vi "PROJEKT-APIR-IMIR.vi"() -> ()   [LabVIEW 2019]
uses:
  <vilib>/addons/Control Design/_Model Construction/Model Typedefs.llb/CD Transfer Function Model (MIMO).ctl
  <vilib>/addons/Control Design/_Model Construction/Model Typedefs.llb/CD General Elements.ctl
  <vilib>/addons/Control Design/_Model Construction/Model Typedefs.llb/CD Transfer Function Model (SISO).ctl
  <vilib>/addons/Control Design/_Model Construction/Data Typedefs.llb/CD MIMO Time Response Data.ctl
  <vilib>/addons/Control Design/_Model Construction/Data Typedefs.llb/CD Plot Types Enum.ctl
  <vilib>/addons/Control Design/_Model Construction/Data Typedefs.llb/CD frequency specs.ctl
  <vilib>/addons/Control Design/_Model Construction/Data Typedefs.llb/CD Time Info.ctl
  <vilib>/addons/Control Design/_Model Conversions/Model Type.llb/Model Conversion SubVI/cd_Convert Transfer Function to State-Space Model.vi
  <vilib>/addons/Control Design/_Frequency Response Analysis/Frequency Response.llb/Frequency Response subVI/cd_Bode (State Space).vi
  <vilib>/addons/Control Design/_Frequency Response Analysis/Frequency Response.llb/Frequency Response subVI/cd_Evaluate at Frequency (State-Space).vi
  <vilib>/addons/Control Design/_Frequency Response Analysis/Frequency Response.llb/Frequency Response subVI/cd_Nyquist (State-Space).vi
  <vilib>/addons/Control Design/_Model Construction/Model Creation.llb/Model Creation SubVI/cd_Create Symbolic Transfer Function Model.vi
  <vilib>/addons/Control Design/_Utility/Model Viewer.llb/Model Viewer SubVI/cd_Draw State-Space Equation (SS).vi
  <vilib>/addons/Control Design/_Utility/Model Viewer.llb/Model Viewer SubVI/cd_Draw Transfer Function Equation (TF).vi
  <vilib>/addons/Control Design/_Model Interconnection/Model Interconnection.llb/Model Interconnection SubVI/cd_Element Multiply Models (TF and Gain).vi
  <vilib>/addons/Control Design/_Time Response Analysis/Time Response.llb/Time Response subVI/cd_Initial Response (State-Space).vi
  <vilib>/addons/Control Design/_Time Response Analysis/Time Response.llb/Time Response subVI/cd_Step Response (State-Space).vi
  <vilib>/addons/Control Design/_Time Response Analysis/Time Response.llb/Time Response subVI/cd_Impulse Response (State-Space).vi
  <vilib>/addons/Control Design/_Time Response Analysis/Time Response.llb/Time Response subVI/cd_Linear Simulation (State-Space).vi
  <vilib>/addons/Control Design/_Time Response Analysis/Time Response.llb/Time Response subVI/cd_Impulse Response (Transfer Function).vi
  <vilib>/addons/Control Design/_Model Construction/NI_LinSys_Model Creation.lvlib
  <vilib>/addons/Control Design/_Utility/NI_CD_Model Viewer.lvlib
  <vilib>/addons/Control Design/_Time Response Analysis/NI_CD_Time Response.lvlib
  <vilib>/addons/Control Design/_Model Conversions/NI_CD_Model Type.lvlib
  <vilib>/addons/Control Design/_Model Construction/NI_LinSys_Data Typedefs.lvlib
  <vilib>/addons/Control Design/_Frequency Response Analysis/NI_CD_Frequency Response.lvlib
  <vilib>/addons/Control Design/_Model Interconnection/NI_CD_Model Interconnection.lvlib
  <vilib>/addons/Control Design/_Model Construction/NI_LinSys_Model Typedefs.lvlib
panel:
  in  "input cluster":T1={"Time"=array[5001 elements], "Outputs Data"=array1x5001x1[5001 elements], "States Data"=array1x5001x2[10002 elements], "plot type"=enum."impulse"} {"States Data" format="%#.6g"; "Outputs Data" format="%#.6g"; "Time" format="%#.6g"}
  in  "Initial Conditions":dbl[](array[numeric])=[0.0, 0.0]
  out "Transfer Function Model":T3={"properties"={"Model name"="System Model", "Input names"=["u0"], "Output names"=["y0"], "Input Delays"=[0.0], "Output Delays"=[0.0], "Sampling Time"=0.0, "Notes"=""}, "transfer function(s)"=[[{"Numerator"=[-1.0], "Denominator"=[3.0, 2.0, 4.0], "delay"=0.0}]]} {"transfer function(s)"."delay" format="%.4f"; "transfer function(s)"."Denominator" format="%#_3g"; "transfer function(s)"."Numerator" format="%#_3g"; "properties"."Sampling Time" format="%#.6p"; "properties"."Output Delays" format="%.4f"; "properties"."Input Delays" format="%.4f"}
  in  "Draw Area Size":cluster{"Width":u32, "Height":u32}={"Width"=117, "Height"=36}
  in  "Origin Drawing":cluster{"x":i16, "y":i16}={"x"=4, "y"=6}
  in  "y":dbl=-9.0 min=-9.0 format="%#_13g"
  in  "stop":bool
  in  "?":T6(tab)=enum."Animacja"
  in  "Masa":dbl=4.0 min=1.0 format="%#_6p"
  in  "Współczynnik tłumienia":dbl=2.0 min=1.0 format="%#_6p"
  in  "Współczynnik sprężystości":dbl=3.0 min=1.0 format="%#_6p"
  out "Equation":picture
  out "Equation 2":picture
  out "Equation 3":picture
  in  "Typ charakterystyki":u16(ring)=2 items=["All in one", "Odpowiedź na skok", "Odpowiedź na impuls", "Odpowiedź na wym. sinusoidalne", "Odpowiedź tylko na warunki początkowe"]
  in  "Siła Przyłożona \"w dół\"":dbl=-1.0 step=0.1 format="%#_6p"
  in  "Wychylenie początkowe":dbl min=0.0 step=0.1 format="%#_6p"
  in  "Prędkość początkowa":dbl min=0.0 step=0.1 format="%#_6p"
  in  "Częstotliwosć źródła":dbl=10.0 caption="Frequency" step=10.0
  out "All 2":cluster{"time":dbl[], dbl[]}[](graph)
  in  "Jednostka czestotliwosci":enum16{"Hz", "rad/s"}(ring)
  in  "Czestotliwosc poczatkowa":dbl=-1.0
  in  "Wartosc czestotliwosci":dbl=4.0 step=0.1
  out "Charakterystyka amplitudowo fazowa":cluster{"W":dbl[], "Magnitude":dbl[]}[](graph)
  out "Charakterystyka fazowo czestotliwosciowa":cluster{"W":dbl[], "Magnitude":dbl[]}[](graph)
  out "Charakterystyka amplitudowo czestotliwosciowa":cluster{"W":dbl[], "Magnitude":dbl[]}[](graph)
  out "Faza":dbl=1.1410674686545497
  out "Wzmocnienie dB":dbl=-68.0421974527826
  out "AMPLITUDE SCALE":dbl
  out "String 2":string
  out "Slide":u8(slide) scale=0.0..100.0
  out "String":string="Odpowiedź na impuls"
  in  "Start/Ponów":bool
  out "?":picture
  in  "STOP":bool
  # "PROGRAM ROZWIĄZUJĄCY MODEL UKŁADU T-M-S"
  # "Program służy do rozwiązywania zadanego układu mechanicznego tłumik-masa-sprężyna.\nWejściem w układzie jest siła F, natomiast odpowiedzią układu jest przesunięcie y.\nW zakładce Transformata Laplaca możemy zadać parametry układu i zobaczyć transmitancje układu po podstawieniu zmiennych. Dodatkowo możemy zobaczyć tam macierze stanów układu.\nW zakładce Wykresy czasowe możemy zadać warunki początkowe oraz siłę, jako wynik utrzymujemy wykresy odpowiedzi na wymuszenie w przestrzeni czasu.\nW zakładce Wykresy częstotliwościowe dostępne są charakterystyki Nyquista (amplitudowo-fazowa) oraz Bodego (amplitudowo-częstotliwościowa & fazowo-częstotliwościowa).\nW zakładce Animacja możemy zobaczyć symulacje układu."
  # "*Dane do programu należy wpisywać używając jednostek SI."
  # "Designed by: M. Waksmundzki, M. Zajda, D. Załóg [Automatyka Przemysłowa i Robotyka]"
  # "TRANSMITANCJA DLA ZADANYCH PARAMETRÓW:"
  # "MACIERZE STANÓW UKŁADU:"
  # "CHARAKTERYSTYKA AMPLITUDOWO-CZĘSTOTLIWOŚCIOWA"
  # "CHARAKTERYSTYKA AMPLITUDOWO-FAZOWA"
  # "CHARAKTERYSTYKA FAZOWO-CZĘSTOTLIWOŚCIOWA"
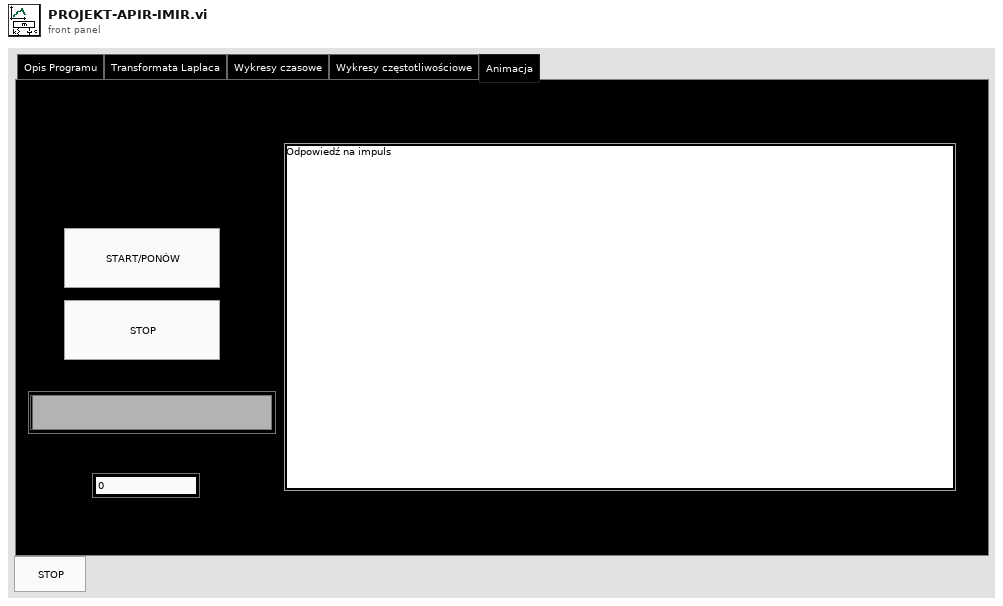
[diagram p1: front panel]
types:
  T1 = typedef "NI_LinSys_Data Typedefs.lvlib/CD MIMO Time Response Data.ctl" = cluster{"Time":dbl[], "Outputs Data":dbl[][][], "States Data":dbl[][][], "plot type":T2}
  T2 = typedef "NI_LinSys_Data Typedefs.lvlib/CD Plot Types Enum.ctl" = enum16{"bode-magnitude", "bode-phase", "nichols", "nyquist", "singular values", "step", "impulse", "initial", "simulation", "nyquist with separation"}
  T3 = typedef "NI_LinSys_Model Typedefs.lvlib/CD Transfer Function Model (MIMO).ctl" = cluster{"properties":T4, "transfer function(s)":T5[][]}
  T4 = typedef "NI_LinSys_Model Typedefs.lvlib/CD General Elements.ctl" = cluster{"Model name":string, "Input names":string[], "Output names":string[], "Input Delays":dbl[], "Output Delays":dbl[], "Sampling Time":dbl, "Notes":string}
  T5 = typedef "NI_LinSys_Model Typedefs.lvlib/CD Transfer Function Model (SISO).ctl" = cluster{"Numerator":dbl[], "Denominator":dbl[], "delay":dbl}
  T6 = enum32{"Opis Programu", "Transformata Laplaca", "Wykresy czasowe", "Wykresy częstotliwościowe", "Animacja"}
  T7 = typedef "NI_LinSys_Data Typedefs.lvlib/CD frequency specs.ctl" = cluster{"Initial frequency":dbl, "Final frequency":dbl, "Minimum number of points":i32, "Frequency Unit":enum16{"Hz", "rad/s"}}
  T8 = typedef "NI_LinSys_Data Typedefs.lvlib/CD Time Info.ctl" = cluster{"t0":dbl, "dt":dbl, "tf":dbl}
  T9 = typedef "NI_LinSys_Model Typedefs.lvlib/CD State Space Model (MIMO).ctl" = cluster{"properties":T4, "A":dbl[][], "B":dbl[][], "C":dbl[][], "D":dbl[][], "StateNames":string[], "Transport Delay":dbl[][]}
  T10 = cluster{string, "Współczynnik sprężystości":dbl}[]
  T11 = typedef "LVBoundsTypeDef.ctl" = cluster{"Width":u32, "Height":u32}
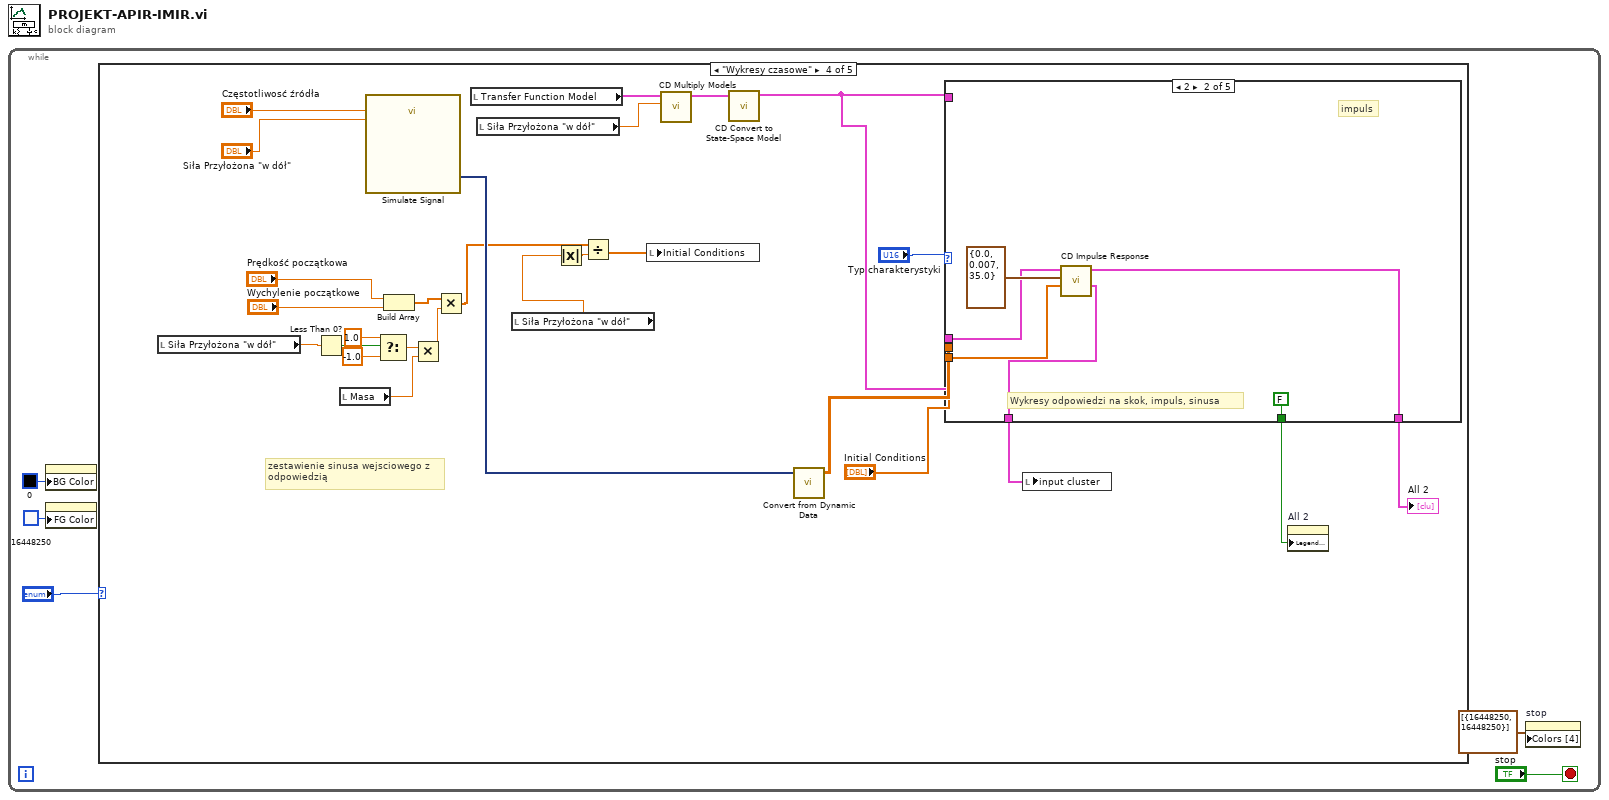
[diagram p0: block diagram]
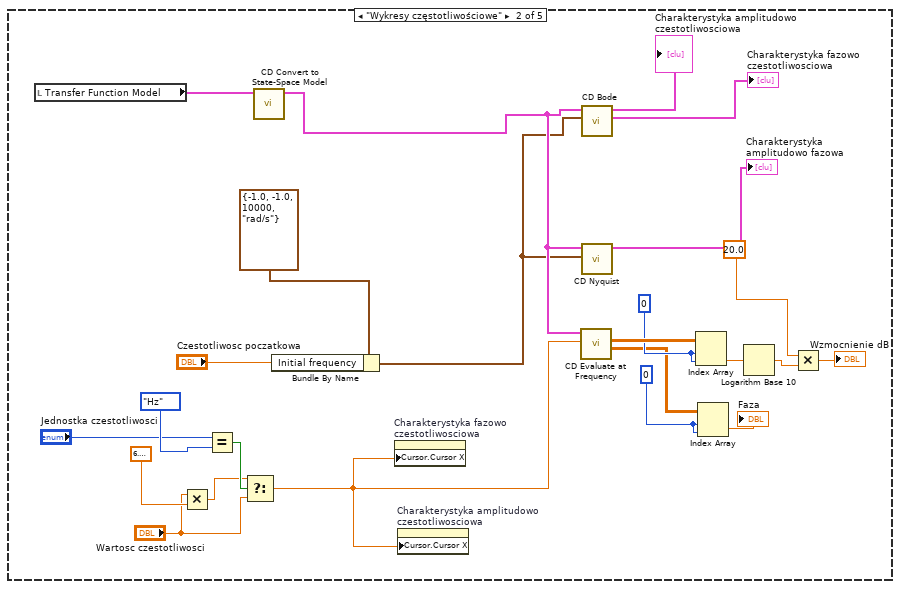
[diagram p3: hidden frame]
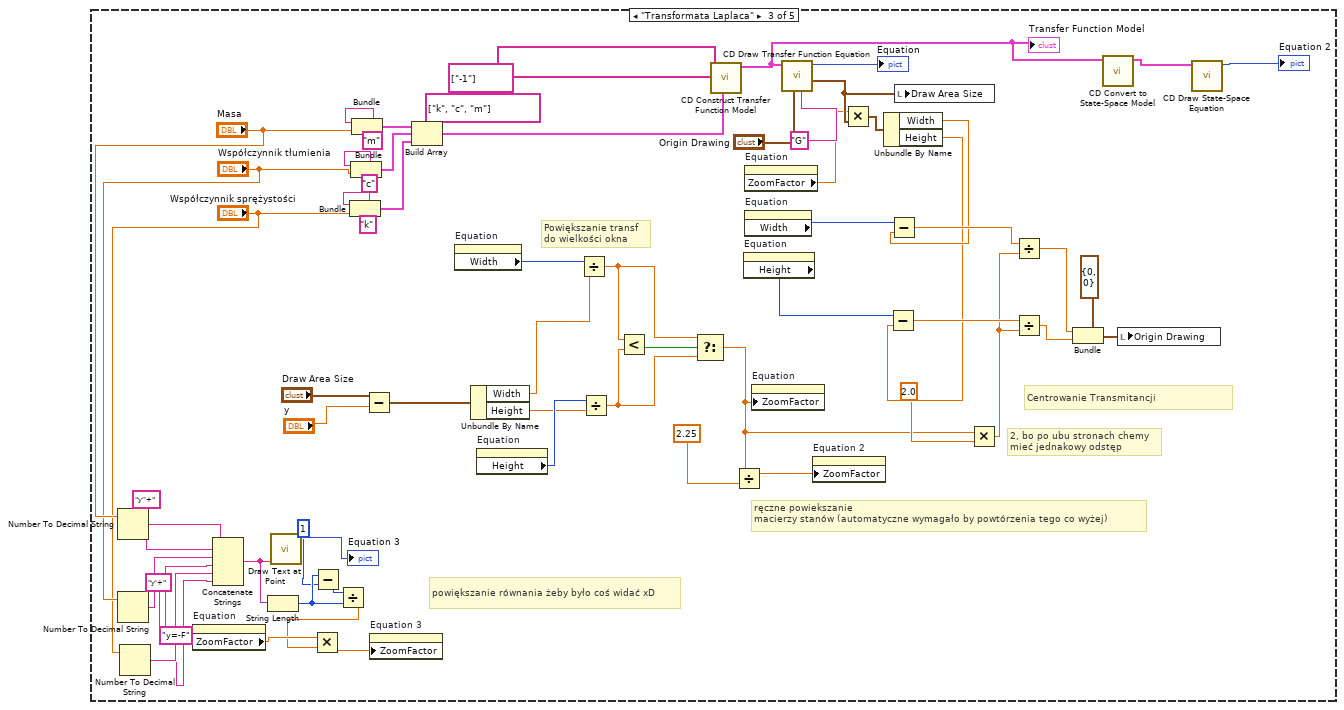
[diagram p4: hidden frame]
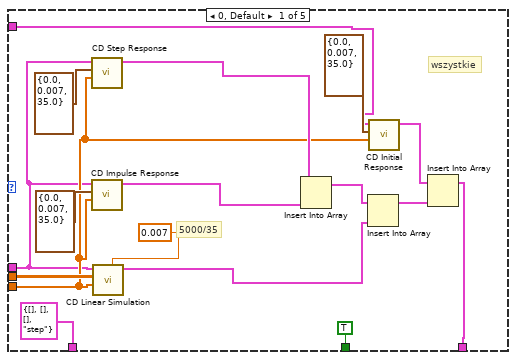
[diagram p5: hidden frame]
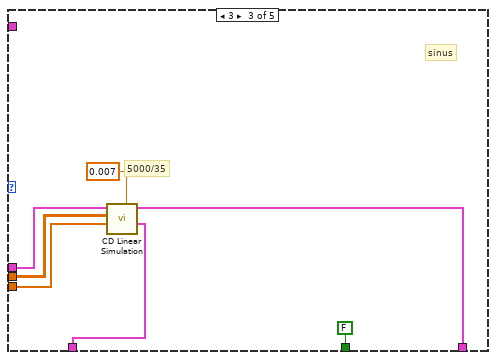
[diagram p6: hidden frame]
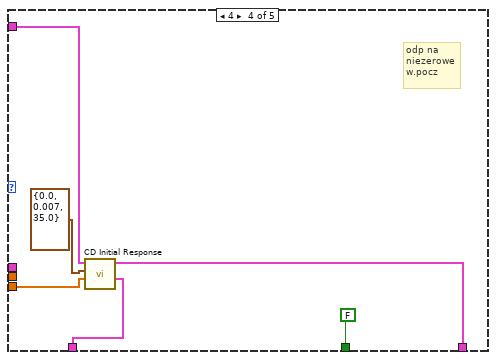
[diagram p7: hidden frame]
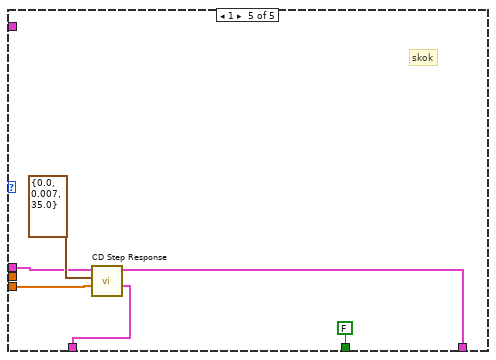
[diagram p8: hidden frame]
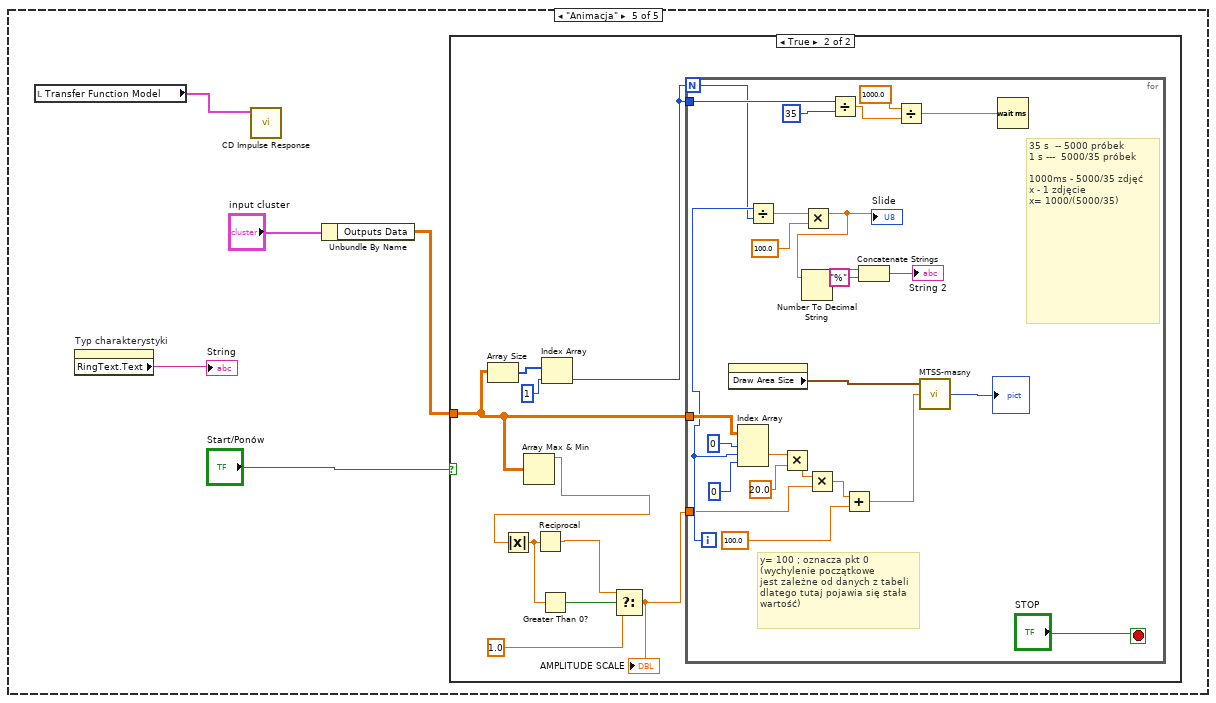
[diagram p9: hidden frame]
diagram:
  n1 = while {
    stop <- "stop" stop-if-true
    n2 = property class="TabCtl (strict)"("BG Color"=u32 0 ("Colors:BG Color")) -> ()  [unwired: 2 in, 2 out]
    n3 = property class="TabCtl (strict)"("FG Color"=u32 16448250 ("Colors:FG Color")) -> ()  [unwired: 2 in, 2 out]
    n4 = case shown="\"Wykresy czasowe\"" "?" {
      frame "Opis Programu", Default {
      }
      frame "Wykresy częstotliwościowe" {
        w25 = 0 ("index (row)")
        w26 = 0 ("index (row)")
        n5 = local read "Transfer Function Model"() -> (w12:T3)
        n6 = Multiply(x="Wartosc czestotliwosci", y=6.283185307179586) -> (x*y=w10:dbl)
        n7 = Equal?(x="Jednostka czestotliwosci", y=enum16{"Hz", "rad/s"}."Hz" ("Frequency Unit")) -> (x = y?=w16:bool)
        n8 = Select(t=w10, s=w16, f="Wartosc czestotliwosci") -> (s? t:f=w11:dbl)
        n9 = call-poly <vilib>:"CD Convert to State-Space Model.vi"("Transfer Function Model"=w12) -> ("State-Space Model"=w13:T9)  [unwired: 9 in, 1 out]
        n10 = Bundle By Name(cluster=T7 {"Initial frequency"=-1.0, "Final frequency"=-1.0, "Minimum number of points"=10000, "Frequency Unit"=enum."rad/s"} ("Frequency Range"), "Initial frequency"="Czestotliwosc poczatkowa") -> (w6:T7)
        n11 = property on="Charakterystyka fazowo czestotliwosciowa" class="XYGraph (strict)"("Cursor.Cursor X"=w11) -> ()  [unwired: 2 in, 2 out]
        n12 = property on="Charakterystyka amplitudowo czestotliwosciowa" class="XYGraph (strict)"("Cursor.Cursor X"=w11) -> ()  [unwired: 2 in, 2 out]
        n13 = call-poly <vilib>:"CD Evaluate at Frequency.vi"("Frequency (rad/s)"=w11, "State-Space Model"=w13) -> ("Phase (deg)"=w24:dbl[][], "Magnitude"=w27:dbl[][])  [unwired: 6 in, 2 out]
        n14 = call-poly <vilib>:"CD Bode.vi"("Frequency Range"=w6, "State-Space Model"=w13) -> ("Bode Phase"=→"Charakterystyka fazowo czestotliwosciowa":cluster{"W":dbl[], "Magnitude":dbl[]}[], "Bode Magnitude"=→"Charakterystyka amplitudowo czestotliwosciowa":cluster{"W":dbl[], "Magnitude":dbl[]}[])  [unwired: 5 in, 3 out]
        n15 = call-poly <vilib>:"CD Nyquist.vi"("Frequency Range"=w6, "State-Space Model"=w13) -> ("Nyquist Plot"=→"Charakterystyka amplitudowo fazowa":cluster{"W":dbl[], "Magnitude":dbl[]}[])  [unwired: 7 in, 2 out]
        n16 = Index Array(array=w27, index (row)=w26, index (col)=w26) -> (element=w21:dbl)
        n17 = Index Array(array=w24, index (row)=w25, index (col)=w25) -> (element=→"Faza":dbl)
        n18 = Logarithm Base 10(1:w21) -> (0:w20:dbl)
        n19 = Multiply(x=20.0, y=w20) -> (x*y=→"Wzmocnienie dB":dbl)
      }
      frame "Transformata Laplaca" {
        # "powiększanie równania żeby było coś widać xD"
        # "ręczne powiekszanie\nmacierzy stanów (automatyczne wymagało by powtórzenia tego co wyżej)"
        # "2, bo po ubu stronach chemy\nmieć jednakowy odstęp"
        # "Powiększanie transf \ndo wielkości okna"
        # "Centrowanie Transmitancji"
        n20 = Number To Decimal String(number="Masa") -> (decimal integer string=w46:string)  [unwired: 1 in]
        n21 = Number To Decimal String(number="Współczynnik tłumienia") -> (decimal integer string=w45:string)  [unwired: 1 in]
        n22 = Number To Decimal String(number="Współczynnik sprężystości") -> (decimal integer string=w43:string)  [unwired: 1 in]
        n23 = property on="Equation" class="Pict"() -> ("ZoomFactor"=w39:sgl)  [unwired: 2 in, 2 out]
        n24 = Concatenate Strings(w46, "y''+", w45, "y'+", w43, "y=-F") -> (w37:string)
        n25 = String Length(string=w37) -> (length=w35:i32)
        n26 = call <vilib>:"Draw Text at Point.vi"("text"=w37) -> ("new picture"=→"Equation 3":picture)  [unwired: 9 in, 1 out]
        n27 = Subtract(x=w35, y=1 ("x")) -> (x-y=w34:i32)
        n28 = Divide(x=w34, y=w35) -> (x/y=w36:dbl)
        n29 = Multiply(x=w39, y=w36) -> (x*y=w38:dbl)
        n30 = Bundle("k", "Współczynnik sprężystości"="Współczynnik sprężystości") -> (w85:cluster{string, "Współczynnik sprężystości":dbl})  [unwired: 1 in]
        n31 = Bundle("c", "Współczynnik tłumienia"="Współczynnik tłumienia") -> (w86:cluster{string, "Współczynnik tłumienia":dbl})  [unwired: 1 in]
        n32 = Bundle("m", "Masa"="Masa") -> (w87:cluster{string, "Masa":dbl})  [unwired: 1 in]
        n33 = Subtract(x="Draw Area Size", y="y") -> (x-y=w65:cluster{"Width":dbl, "Height":dbl})
        n34 = property on="Equation 3" class="Pict"("ZoomFactor"=w38) -> ()  [unwired: 2 in, 2 out]
        n35 = Build Array(w87, w86, w85) -> (w84:T10)
        n36 = property on="Equation" class="Pict"() -> ("Width"=w62:u32)  [unwired: 2 in, 2 out]
        n37 = Unbundle By Name(w65) -> ("Width"=w61:dbl, "Height"=w63:dbl)
        n38 = property on="Equation" class="Pict"() -> ("Height"=w64:u32)  [unwired: 2 in, 2 out]
        n39 = Divide(x=w62, y=w61) -> (x/y=w59:dbl)
        n40 = Divide(x=w64, y=w63) -> (x/y=w58:dbl)
        n41 = Less?(x=w59, y=w58) -> (x < y?=w60:bool)
        n42 = Select(t=w59, s=w60, f=w58) -> (s? t:f=w40:dbl)
        n43 = call-poly <vilib>:"CD Construct Transfer Function Model.vi"("Variables"=w84, "Symbolic Denominator"=string[] ["k", "c", "m"], "Symbolic Numerator"=string[] ["-1"]) -> ("Transfer Function Model"=w52:T3)  [unwired: 7 in, 1 out]
        "Transfer Function Model" <- w52
        n44 = Divide(x=w40, y=2.25) -> (x/y=w49:dbl)
        n45 = property on="Equation" class="Pict"() -> ("Height"=w75:u32)  [unwired: 2 in, 2 out]
        n46 = property on="Equation" class="Pict"() -> ("ZoomFactor"=w53:sgl)  [unwired: 2 in, 2 out]
        n47 = property on="Equation" class="Pict"() -> ("Width"=w76:u32)  [unwired: 2 in, 2 out]
        n48 = property on="Equation" class="Pict"("ZoomFactor"=w40) -> ()  [unwired: 2 in, 2 out]
        n49 = call-poly <vilib>:"CD Draw Transfer Function Equation.vi"("Function Name (empty)"="G", "Origin"="Origin Drawing", "Transfer Function Model"=w52) -> ("Draw Area Size"=w55:cluster{"Width":u32, "Height":u32}, "Equation"=→"Equation":picture)  [unwired: 6 in, 1 out]
        n50 = property on="Equation 2" class="Pict"("ZoomFactor"=w49) -> ()  [unwired: 2 in, 2 out]
        n51 = Multiply(x=w53, y=w55) -> (x*y=w69:cluster{"Width":sgl, "Height":sgl})
        n52 = Unbundle By Name(w69) -> ("Width"=w72:sgl, "Height"=w70:sgl)
        n53 = Subtract(x=w75, y=w70) -> (x-y=w71:sgl)
        n54 = Subtract(x=w76, y=w72) -> (x-y=w73:sgl)
        n55 = local write "Draw Area Size"(w55) -> ()
        n56 = Multiply(x=w40, y=2.0) -> (x*y=w67:dbl)
        n57 = Divide(x=w73, y=w67) -> (x/y=w78:dbl)
        n58 = Divide(x=w71, y=w67) -> (x/y=w77:dbl)
        n59 = Bundle(cluster=cluster{"x":i16, "y":i16} {"x"=0, "y"=0} ("Origin"), "x"=w78, "y"=w77) -> (w54:cluster{"x":i16, "y":i16})
        n60 = call-poly <vilib>:"CD Convert to State-Space Model.vi"("Transfer Function Model"=w52) -> ("State-Space Model"=w51:T9)  [unwired: 9 in, 1 out]
        n61 = local write "Origin Drawing"(w54) -> ()
        n62 = call-poly <vilib>:"CD Draw State-Space Equation.vi"("State-Space Model"=w51) -> ("Equation"=→"Equation 2":picture)  [unwired: 8 in, 2 out]
      }
      frame "Wykresy czasowe" {
        # "zestawienie sinusa wejsciowego z\nodpowiedzią"
        # "Wykresy odpowiedzi na skok, impuls, sinusa"
        n63 = local read "Siła Przyłożona \"w dół\""() -> (w101:dbl)
        n64 = Less Than 0?(x=w101) -> (x < 0?=w100:bool)
        n65 = local read "Masa"() -> (w90:dbl)
        n66 = call "Simulate Signal"("Frequency"="Częstotliwosć źródła", "Amplitude"="Siła Przyłożona \"w dół\"") -> ("Sine"=w114:dynamicdata)  [unwired: 12 in, 1 out]
        n67 = Select(t=1.0, s=w100, f=-1.0) -> (s? t:f=w97:dbl)
        n68 = Build Array("Prędkość początkowa", "Wychylenie początkowe") -> (w102:dbl[])
        n69 = Multiply(x=w97, y=w90) -> (x*y=w91:dbl)
        n70 = Multiply(x=w102, y=w91) -> (x*y=w95:dbl[])
        n71 = local read "Transfer Function Model"() -> (w105:T3)
        n72 = local read "Siła Przyłożona \"w dół\""() -> (w103:dbl)
        n73 = local read "Siła Przyłożona \"w dół\""() -> (w94:dbl)
        n74 = Absolute Value(x=w94) -> (abs(x)=w93:dbl)
        n75 = Divide(x=w95, y=w93) -> (x/y=w96:dbl[])
        n76 = local write "Initial Conditions"(w96) -> ()
        n77 = call-poly <vilib>:"CD Multiply Models.vi"("Gain"=w103, "Model 1"=w105) -> ("Model Out"=w92:T3)  [unwired: 8 in, 1 out]
        n78 = call-poly <vilib>:"CD Convert to State-Space Model.vi"("Transfer Function Model"=w92) -> ("State-Space Model"=w104:T9)  [unwired: 9 in, 1 out]
        n79 = call "Convert from Dynamic Data"("Dynamic Data Type"=w114) -> ("Array"=w112:dbl[][])  [unwired: 3 in]
        n80 = case shown="2" "Typ charakterystyki" {
          tunnel: w112 -> [w128 _ w144 _ _]
          tunnel: w104 -> [w123 w138 w145 _ w157]
          tunnel: "Initial Conditions" -> [w124 w137 w143 w152 w156]
          tunnel: [w120 w136 w142 w150 w155] -> w110
          tunnel: w104 -> [w119 _ _ w149 _]
          tunnel: [TRUE ("Scale Legend:Visible") FALSE ("Scale Legend:Visible") FALSE ("Scale Legend:Visible") FALSE ("Scale Legend:Visible") FALSE ("Scale Legend:Visible")] -> w109
          tunnel: [T1 {"Time"=[], "Outputs Data"=[], "States Data"=[], "plot type"=enum."step"} ("Step Response Data") w134 w140 w147 w153] -> w108
          frame 0, Default {
            # "wszystkie"
            # "5000/35"
            n81 = call-poly <vilib>:"CD Step Response.vi"("Initial Conditions"=w124, "Time Range"=T8 {"t0"=0.0, "dt"=0.007, "tf"=35.0}, "State-Space Model"=w123) -> ("Step Response Graph"=w130:cluster{"time":dbl[], dbl[]}[])  [unwired: 5 in, 3 out]
            n82 = call-poly <vilib>:"CD Impulse Response.vi"("Initial Conditions"=w124, "Time Range"=T8 {"t0"=0.0, "dt"=0.007, "tf"=35.0}, "State-Space Model"=w123) -> ("Impulse Response Graph"=w131:cluster{"time":dbl[], dbl[]}[])  [unwired: 5 in, 3 out]
            n83 = call-poly <vilib>:"CD Linear Simulation.vi"("Delta t"=0.007, "Initial Conditions"=w124, "Inputs"=w128, "State-Space Model"=w123) -> ("Simulation Graph"=w133:cluster{"time":dbl[], dbl[]}[])  [unwired: 4 in, 3 out]
            n84 = Insert Into Array(array=w130, new element=w131) -> (w132:cluster{"time":dbl[], dbl[]}[])  [unwired: 1 in]
            n85 = Insert Into Array(array=w132, new element=w133) -> (w122:cluster{"time":dbl[], dbl[]}[])  [unwired: 1 in]
            n86 = call-poly <vilib>:"CD Initial Response.vi"("Initial Conditions"=w124, "Time Range"=T8 {"t0"=0.0, "dt"=0.007, "tf"=35.0}, "State-Space Model"=w119) -> ("Initial Response Graph"=w121:cluster{"time":dbl[], dbl[]}[])  [unwired: 5 in, 3 out]
            n87 = Insert Into Array(array=w121, new element=w122) -> (w120:cluster{"time":dbl[], dbl[]}[])  [unwired: 1 in]
          }
          frame 2 {
            # "impuls"
            n88 = call-poly <vilib>:"CD Impulse Response.vi"("Initial Conditions"=w137, "Time Range"=T8 {"t0"=0.0, "dt"=0.007, "tf"=35.0}, "State-Space Model"=w138) -> ("Impulse Response Data"=w134:T1, "Impulse Response Graph"=w136:cluster{"time":dbl[], dbl[]}[])  [unwired: 5 in, 2 out]
          }
          frame 3 {
            # "sinus"
            # "5000/35"
            n89 = call-poly <vilib>:"CD Linear Simulation.vi"("Delta t"=0.007, "Initial Conditions"=w143, "Inputs"=w144, "State-Space Model"=w145) -> ("Simulation Data"=w140:T1, "Simulation Graph"=w142:cluster{"time":dbl[], dbl[]}[])  [unwired: 4 in, 2 out]
          }
          frame 4 {
            # "odp na\nniezerowe\nw.pocz"
            n90 = call-poly <vilib>:"CD Initial Response.vi"("Initial Conditions"=w152, "Time Range"=T8 {"t0"=0.0, "dt"=0.007, "tf"=35.0}, "State-Space Model"=w149) -> ("Initial Response Data"=w147:T1, "Initial Response Graph"=w150:cluster{"time":dbl[], dbl[]}[])  [unwired: 5 in, 2 out]
          }
          frame 1 {
            # "skok"
            n91 = call-poly <vilib>:"CD Step Response.vi"("Initial Conditions"=w156, "Time Range"=T8 {"t0"=0.0, "dt"=0.007, "tf"=35.0}, "State-Space Model"=w157) -> ("Step Response Data"=w153:T1, "Step Response Graph"=w155:cluster{"time":dbl[], dbl[]}[])  [unwired: 5 in, 2 out]
          }
        }
        "All 2" <- w110
        n92 = local write "input cluster"(w108) -> ()
        n93 = property on="All 2" class="XYGraph (strict)"("Legend Visible"=w109) -> ()  [unwired: 2 in, 2 out]
      }
      frame "Animacja" {
        n94 = local read "Transfer Function Model"() -> (w163:T3)
        n95 = property on="Typ charakterystyki" class="Ring (strict)"() -> ("RingText.Text"=→"String":string)  [unwired: 2 in, 2 out]
        n96 = call-poly <vilib>:"CD Impulse Response.vi"("Transfer Function Model"=w163) -> ()  [unwired: 8 in, 3 out]
        n97 = Unbundle By Name("input cluster") -> ("Outputs Data"=w162:dbl[][][])
        n98 = case shown="True" "Start/Ponów" {
          tunnel: w162 -> [_ w166]
          frame False {
          }
          frame True {
            n99 = Array Size(array=w166) -> (size(s)=w173:i32[])
            n100 = Array Max & Min(array=w166) -> (max value=w165:dbl)  [unwired: 3 out]
            n101 = Absolute Value(x=w165) -> (abs(x)=w167:dbl)
            n102 = Reciprocal(x=w167) -> (1/x=w169:dbl)
            n103 = Greater Than 0?(x=w167) -> (x > 0?=w170:bool)
            n104 = Index Array(array=w173, index=1) -> (element=w171:i32)
            n105 = Select(t=w169, s=w170, f=1.0) -> (s? t:f=w164:dbl)
            "AMPLITUDE SCALE" <- w164
            n106 = for {
              N: w171 -> [w184]
              tunnel: w166 -> [w197]
              tunnel: w171 -> [w191]
              tunnel: w164 -> [w174]
              i -> [w185]
              stop <- "STOP" stop-if-true
              # "y= 100 ; oznacza pkt 0 \n(wychylenie początkowe \njest zależne od danych z tabeli\ndlatego tutaj pojawia się stała \nwartość)"
              # "35 s  -- 5000 próbek\n1 s ---  5000/35 próbek\n\n1000ms - 5000/35 zdjęć \nx - 1 zdjęcie\nx= 1000/(5000/35)"
              n107 = property class="Pict"() -> ("Draw Area Size"=w199:T11)  [unwired: 2 in, 2 out]
              n108 = Index Array(array=w197, index (dim 0)=0 ("index (page)"), index (dim 1)=w185, index (dim 2)=0 ("disabled index (col)")) -> (element=w194:dbl)
              n109 = Divide(x=w185, y=w184) -> (x/y=w183:dbl)
              n110 = Multiply(x=w194, y=20.0) -> (x*y=w176:dbl)
              n111 = Multiply(x=w183, y=100.0) -> (x*y=w181:dbl)
              "Slide" <- w181
              n112 = Number To Decimal String(number=w181) -> (decimal integer string=w180:string)  [unwired: 1 in]
              n113 = Multiply(x=w176, y=w174) -> (x*y=w175:dbl)
              n114 = Divide(x=w191, y=35 ("x")) -> (x/y=w189:dbl)
              n115 = Add(x=w175, y=100.0) -> (x+y=w177:dbl)
              n116 = Concatenate Strings(w180, "%" ("string")) -> (→"String 2":string)
              n117 = Divide(x=1000.0, y=w189) -> (x/y=w188:dbl)
              n118 = call "MTSS-masny.vi"("h"=w177, "frame size"=w199) -> ("Pic out"=→"?":picture)  [unwired: 1 in]
              n119 = Wait (ms)(milliseconds to wait=w188) -> ()  [unwired: 1 out]
            }
          }
        }
      }
    }
    n120 = property on="stop" class="Bool"("Colors [4]"=cluster{u32, u32}[] [{16448250, 16448250}]) -> ()  [unwired: 2 in, 2 out]
  }
